vi "Tree Expand.vi"(0 "Tree Reference In":refnum<vi>, 2 "Tag To Expand":string, 5 "error in (no error)":errorcluster, 9 "Entire Tree (T)":bool=TRUE) -> (14 "Tree Reference Out":refnum<vi>, 19 "error out":errorcluster)   [LabVIEW 2012, in "QuickVIew.lvlib"]
doc: "Expands the entire tree"
uses:
  QuickVIew.lvlib
panel:
  # "VI INPUTS"
  # "VI OUTPUTS"
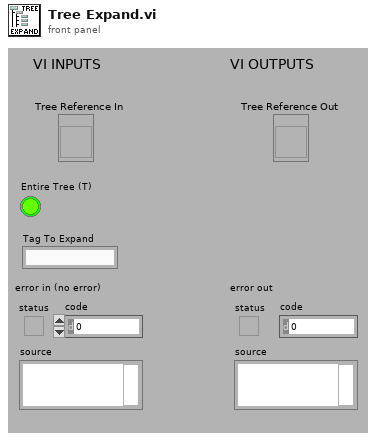
[diagram p1: front panel]
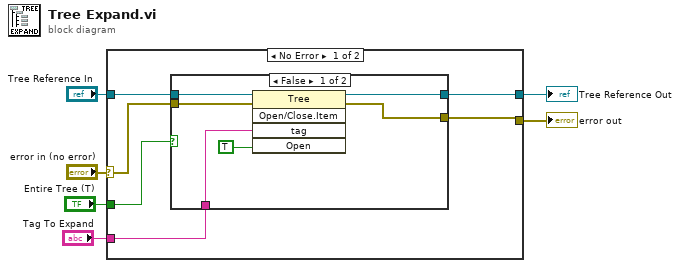
[diagram p0: block diagram]
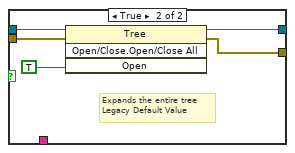
[diagram p2: hidden frame]
diagram:
  n1 = case shown="No Error" "error in (no error)" {
    selector: "error in (no error)" -> [w9 w24]
    tunnel: "Tree Reference In" -> [w10 w25]
    tunnel: [w12 w25] -> w5
    tunnel: [w11 w24] -> w4
    tunnel: "Entire Tree (T)" -> [w8 _]
    tunnel: "Tag To Expand" -> [w7 _]
    frame No Error {
      n2 = case shown="False" w8 {
        tunnel: [w17 w23] -> w12
        tunnel: [w13 w22] -> w11
        tunnel: w10 -> [w18 w21]
        tunnel: w9 -> [w14 w20]
        tunnel: w7 -> [w16 _]
        frame False {
          n3 = invoke class="Tree" method="Open/Close.Item"(reference=w18, error in=w14, "tag"=w16, "Open"=TRUE ("Open?")) -> (reference out=w17:refnum<vi>, error out=w13:errorcluster)  [unwired: 1 in, 3 out]
        }
        frame True {
          # "Expands the entire tree\nLegacy Default Value"
          n4 = invoke class="Tree" method="Open/Close.Open/Close All"(reference=w21, error in=w20, "Open"=TRUE ("Delete Children")) -> (reference out=w23:refnum<vi>, error out=w22:errorcluster)  [unwired: 1 in, 2 out]
        }
      }
    }
    frame Error {
    }
  }
  "Tree Reference Out" <- w5
  "error out" <- w4
